vi "sg Set PSK.vi"(0 "device":i32, 1 "filterAlpha":dbl, 2 "symbolCount":i32, 5 "symbolRate":dbl, 7 "modType":u32(ring) items=["sgModBPSK"=0, "sgModDBPSK"=1, "sgModQPSK"=2, "sgModDQPSK"=3, "sgModOQPSK"=4, "sgModPI4DQPSK"=5, "sgMod8PSK"=6, "sgModD8PSK"=7, "sgMod16PSK"=8, "sgMod16QAM"=9, "sgMod64QAM"=10, "sgMod256QAM"=11, "sgMod8VSB"=20], 9 "filterType":u32(ring) items=["sgRaisedCosine", "sgRootRaisedCosine", "sgGaussian", "sgNone"], 11 "error in (no error)":errorcluster, 12 "symbols":i32) -> (4 "function return":u32(ring), 14 "symbols out":i32, 15 "error out":errorcluster)   [LabVIEW 2014, in "VSG25A.lvlib"]
doc: "SG_API sgStatus sgSetPSK(int device, double symbolRate, sgModulationType modType,\n sgFilterType filterType, double filterAlpha, int *symbols, int symbolCount);"
uses:
  VSG25A.lvlib
  sg_api.dll
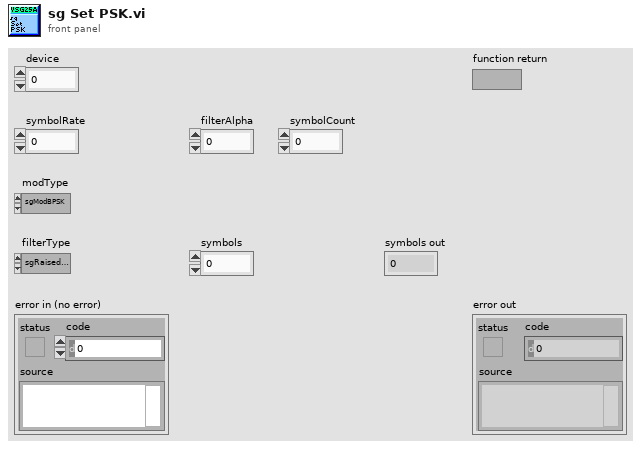
[diagram p1: front panel]
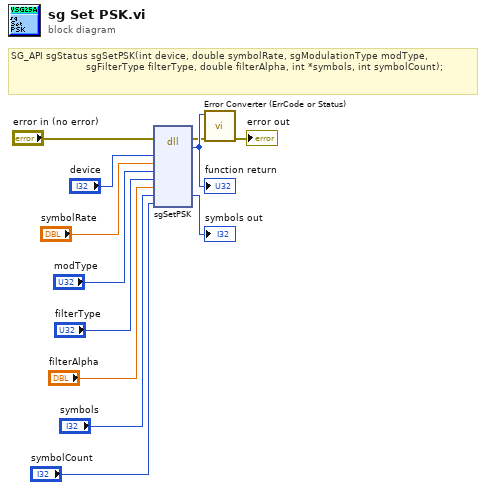
[diagram p0: block diagram]
diagram:
  # "SG_API sgStatus sgSetPSK(int device, double symbolRate, sgModulationType modType,\n                         sgFilterType filterType, double filterAlpha, int *symbols, int symbolCount);"
  n1 = dll-call lib="C:/Users/M_LAPTOP/Desktop/Labview/practice/VSG25A/sg_lib/sg_api.*" fn="sgSetPSK"(error in="error in (no error)", "device"="device", "symbolRate"="symbolRate", "modType"="modType", "filterType"="filterType", "filterAlpha"="filterAlpha", "symbols"="symbols", "symbolCount"="symbolCount") -> (error out=w2:errorcluster, w12:u32, "symbols"=→"symbols out":i32)  [unwired: 8 in, 1 out]
  "function return" <- w12
  n2 = call "Error Converter (ErrCode or Status).vi"("error in (no error)"=w2, "error code"=w12) -> ("error out"=→"error out":errorcluster)  [unwired: 9 in]
